vi "gps.vi"() -> ()   [LabVIEW 2020]
uses:
  <vilib>/Instr/_visa.llb/VISA Configure Serial Port (Instr).vi
panel:
  in  "COM":refnum<visa-resource-name>="COM7"
  in  "error in (no error)":errorcluster caption="에러 입력(에러 없음)"
  out "gga":string
  out "rmc":string
  out "vtg":string
  out "GGA cluster":T1
  out "RMC cluster":T2
  out "VTG cluster":T3
  out "TM_X(lat)":dbl format="%-#_10g M"
  out "TM_Y(long)":dbl format="%-#_10g M"
  out "Heading_T":dbl
  out "Heading_M":dbl
  out "F9P_Data_GPGGA_Raw":string
  out "GPS_KHP":dbl
  out "TM Current":cluster{dbl[], dbl[]}[](array[cluster])
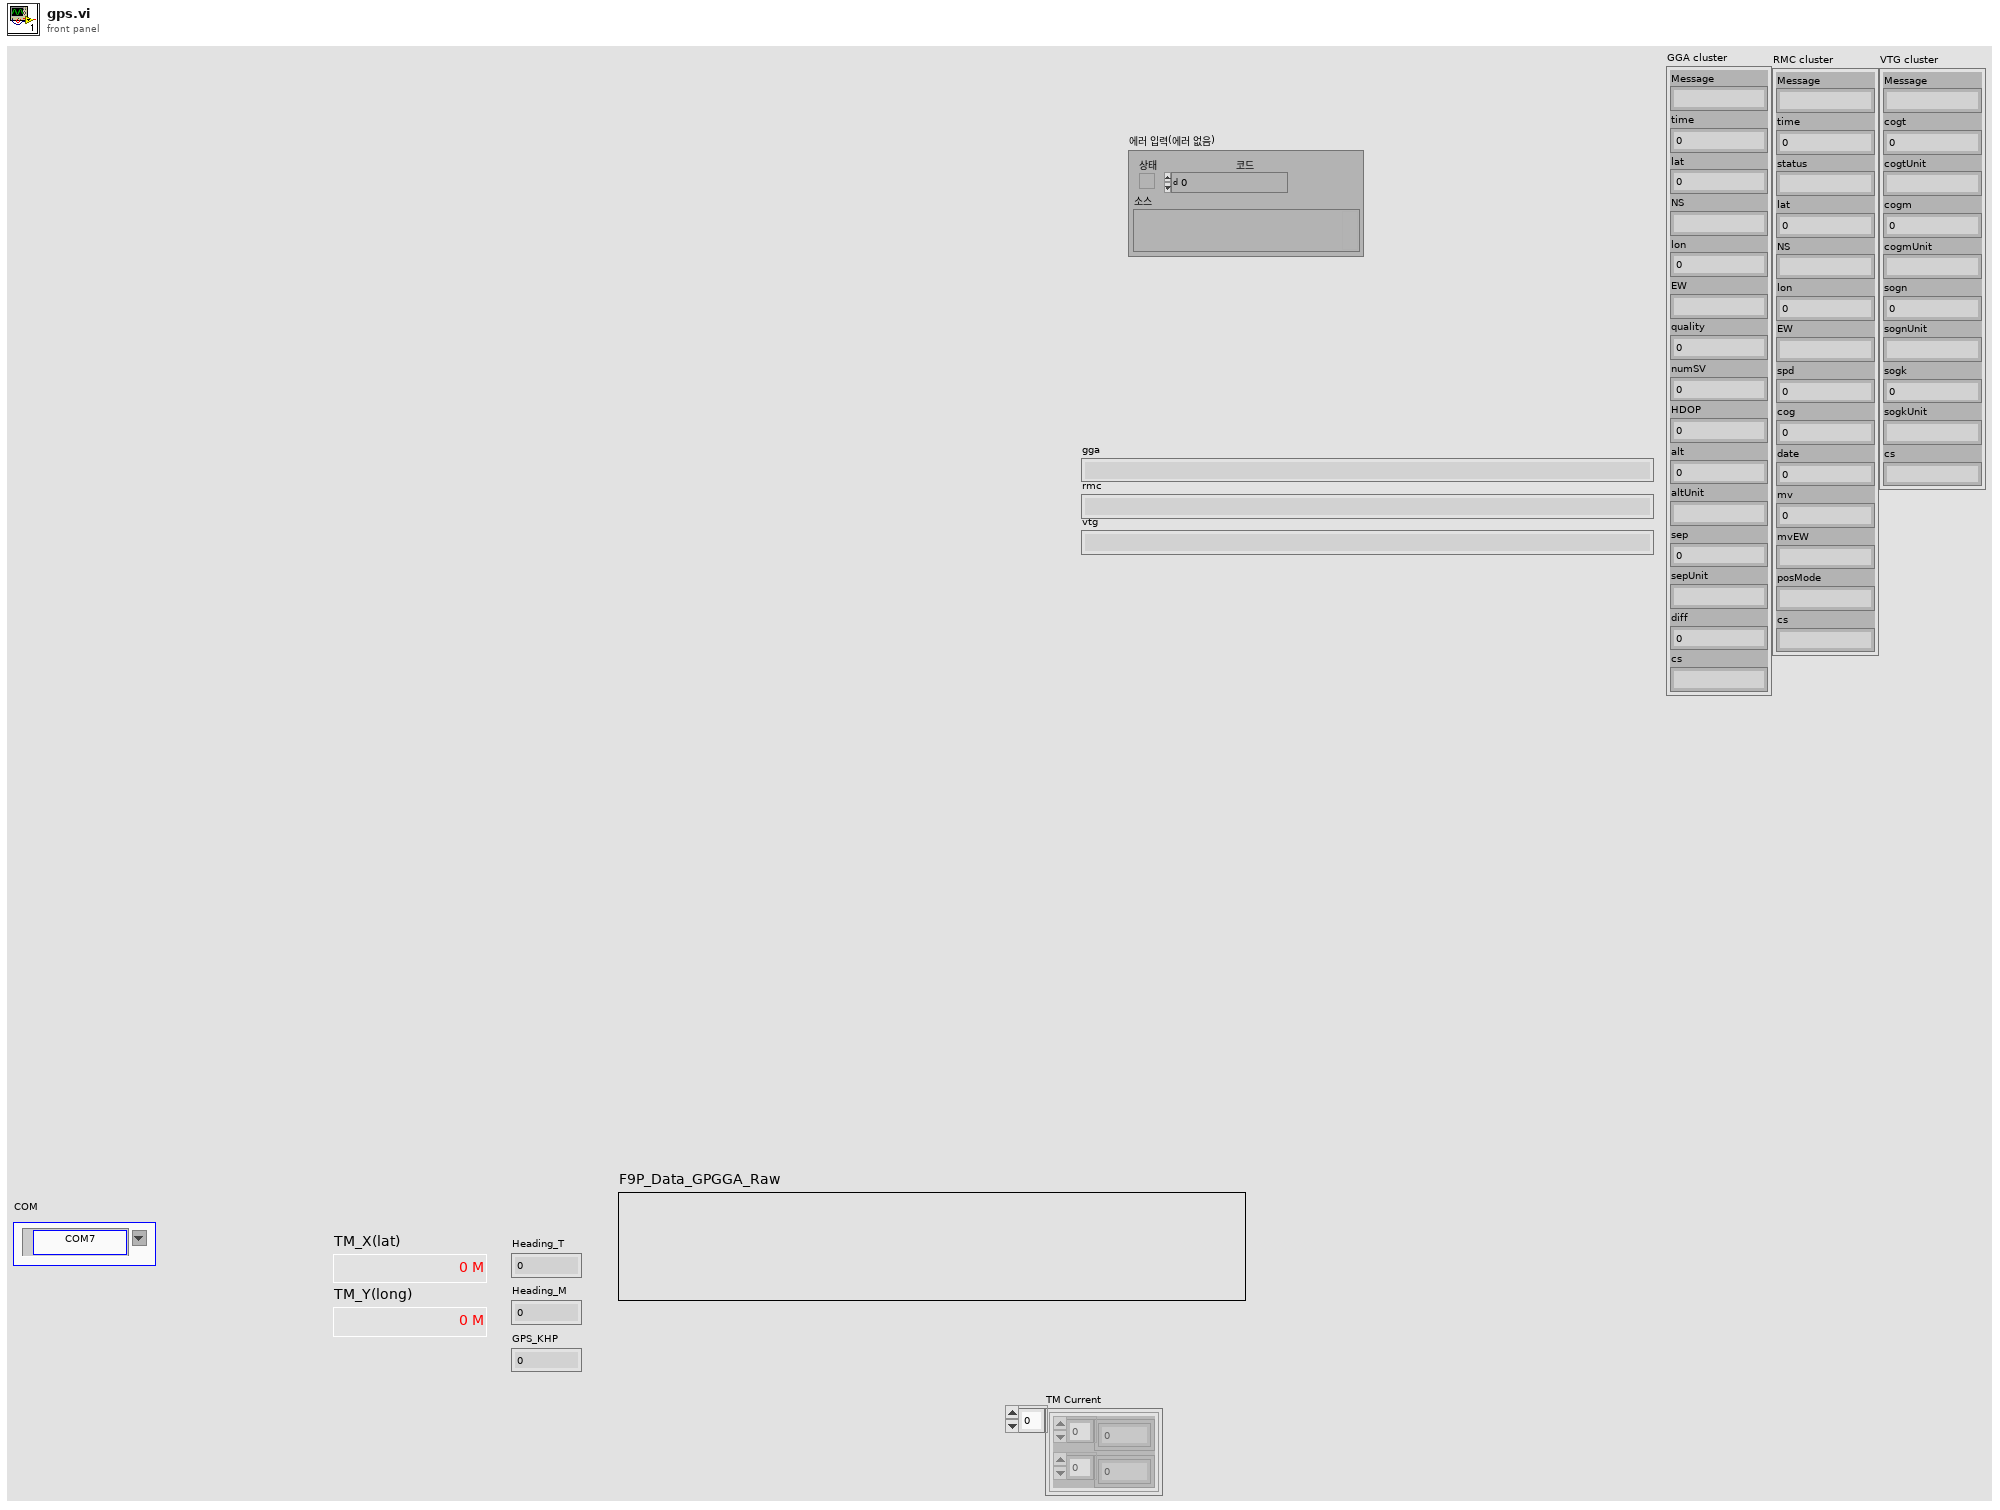
[diagram p1: front panel]
types:
  T1 = cluster{"Message":string, "time":dbl, "lat":dbl, "NS":string, "lon":dbl, "EW":string, "quality":u8, "numSV":u8, "HDOP":dbl, "alt":dbl, "altUnit":string, "sep":dbl, "sepUnit":string, "diff":i32, "cs":string}
  T2 = cluster{"Message":string, "time":dbl, "status":string, "lat":dbl, "NS":string, "lon":dbl, "EW":string, "spd":dbl, "cog":dbl, "date":u32, "mv":dbl, "mvEW":string, "posMode":string, "cs":string}
  T3 = cluster{"Message":string, "cogt":dbl, "cogtUnit":string, "cogm":dbl, "cogmUnit":string, "sogn":dbl, "sognUnit":string, "sogk":dbl, "sogkUnit":string, "cs":string}
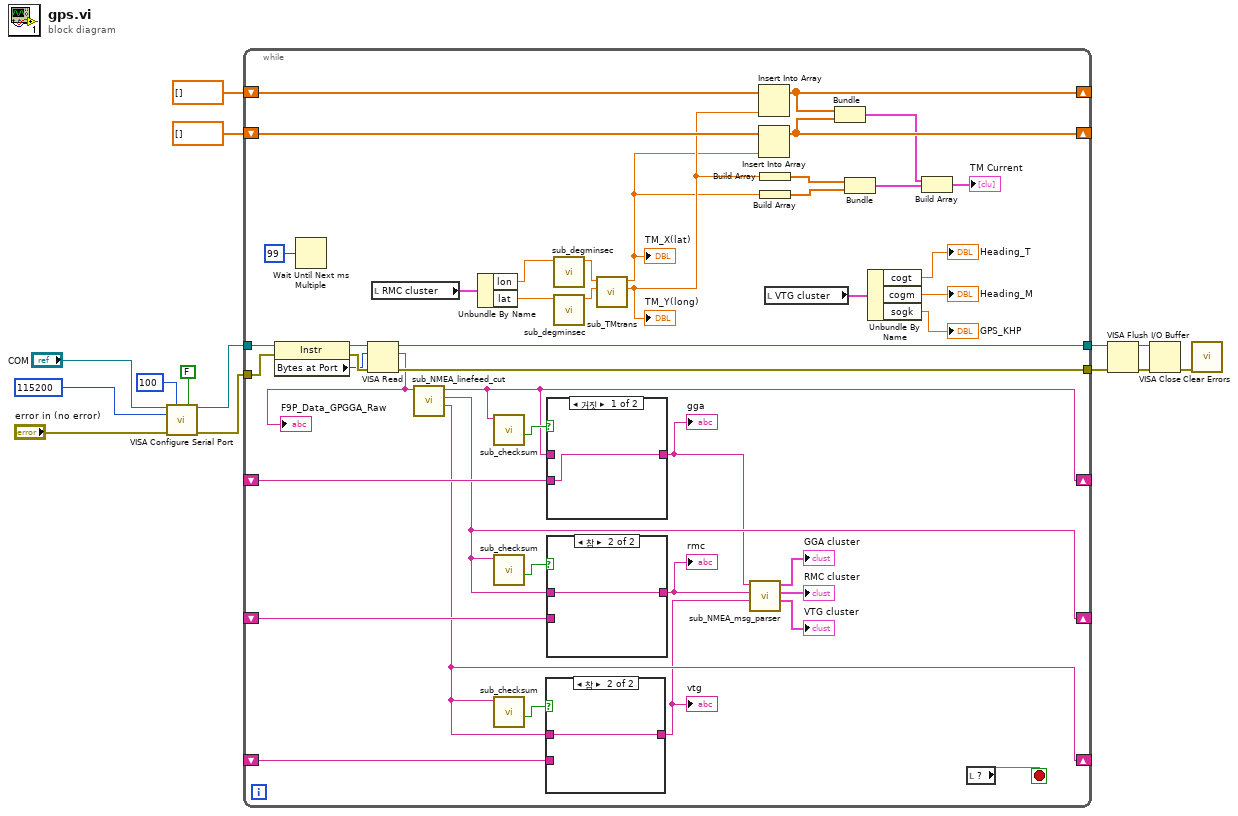
[diagram p0: block diagram]
diagram:
  n1 = call-poly "VISA Configure Serial Port"("VISA resource name"="COM", "timeout (10sec)"=u32 100, "Enable Termination\nChar (T)"=FALSE ("Enable Termination\nChar (T)"), "baud rate (9600)"=u32 115200, "error in (no error)"="error in (no error)") -> ("VISA resource name out"=w13:refnum<visa-resource-name>, "error out"=w12:errorcluster)  [unwired: 9 in]
  n2 = while {
    tunnel: w13 -> [w56]
    tunnel: w12 -> [w55]
    tunnel: [w58] -> w11
    tunnel: [w57] -> w10
    shift-right: [w45] -> _
    shift-left: _ -> [w50]
    shift-right: [w43] -> _
    shift-left: _ -> [w48]
    shift-right: [w44] -> _
    shift-left: _ -> [w46]
    shift-right: [w24] -> _
    shift-left: dbl[] [] -> [w26]
    shift-right: [w23] -> _
    shift-left: dbl[] [] -> [w25]
    stop <- w31 stop-if-true
    n3 = property class="Instr"(reference=w56, error in=w55) -> (reference out=w54:refnum<visa-resource-name>, error out=w53:errorcluster, "Bytes at Port"=w52:u32)
    n4 = Wait Until Next ms Multiple(millisecond multiple=u32 99 ("ms 배수")) -> ()  [unwired: 1 out]
    n5 = VISA Read(VISA resource name=w54, byte count=w52, error in (no error)=w53) -> (VISA resource name out=w58:refnum<visa-resource-name>, read buffer=w15:string, error out=w57:errorcluster)  [unwired: 1 out]
    "F9P_Data_GPGGA_Raw" <- w15
    n6 = local read "RMC cluster"() -> (w29:T2)
    n7 = call "sub_NMEA_linefeed_cut.vi"("GPS raw data buffer"=w15) -> ("GNVTG"=w44:string, "GNRMC"=w43:string, "GNGGA ($제거 문자열)"=w45:string)  [unwired: 8 in]
    n8 = Unbundle By Name(w29) -> ("lon"=w33:dbl, "lat"=w34:dbl)
    n9 = call "sub_checksum.vi"("NMEA String (~\\n이전)"=w45) -> ("equal?"=w51:bool)  [unwired: 6 in, 2 out]
    n10 = call "sub_checksum.vi"("NMEA String (~\\n이전)"=w43) -> ("equal?"=w49:bool)  [unwired: 6 in, 2 out]
    n11 = call "sub_checksum.vi"("NMEA String (~\\n이전)"=w44) -> ("equal?"=w47:bool)  [unwired: 6 in, 2 out]
    n12 = case shown="참" w47 {
      tunnel: [w60 w61] -> w40
      tunnel: w44 -> [_ w61]
      tunnel: w46 -> [w60 _]
      frame False {
      }
      frame True {
      }
    }
    "vtg" <- w40
    n13 = case shown="거짓" w51 {
      tunnel: [w64 w65] -> w42
      tunnel: w45 -> [_ w65]
      tunnel: w50 -> [w64 _]
      frame False {
      }
      frame True {
      }
    }
    "gga" <- w42
    n14 = case shown="참" w49 {
      tunnel: [w62 w63] -> w41
      tunnel: w43 -> [_ w63]
      tunnel: w48 -> [w62 _]
      frame False {
      }
      frame True {
      }
    }
    "rmc" <- w41
    n15 = call "sub_degminsec.vi"("경위도 (lon, lat)"=w33) -> ("도 (degree)"=w35:dbl)  [unwired: 9 in, 1 out]
    n16 = call "sub_degminsec.vi"("경위도 (lon, lat)"=w34) -> ("도 (degree)"=w36:dbl)  [unwired: 9 in, 1 out]
    n17 = call "sub_TMtrans.vi"("위도(lat)_Deg"=w36, "경도(lon)_Deg"=w35) -> ("TM_Y(long)"=w17:dbl, "TM_X(lat)"=w16:dbl)  [unwired: 8 in]
    "TM_X(lat)" <- w16
    "TM_Y(long)" <- w17
    n18 = call "sub_NMEA_msg_parser.vi"("VTG String ($이후~\\n이전)"=w40, "RMC String ($이후~\\n이전)"=w41, "GGA String ($이후~\\n이전)"=w42) -> ("VTG cluster"=→"VTG cluster":T3, "RMC cluster"=→"RMC cluster":T2, "GGA cluster"=→"GGA cluster":T1)  [unwired: 6 in]
    n19 = Insert Into Array(array=w26, new element=w17) -> (w24:dbl[])  [unwired: 1 in]
    n20 = Insert Into Array(array=w25, new element=w16) -> (w23:dbl[])  [unwired: 1 in]
    n21 = Build Array(w17) -> (w22:dbl[])
    n22 = Build Array(w16) -> (w21:dbl[])
    n23 = local read "VTG cluster"() -> (w32:T3)
    n24 = Bundle(w24, w23) -> (w19:cluster{dbl[], dbl[]})  [unwired: 1 in]
    n25 = Bundle(w22, w21) -> (w20:cluster{dbl[], dbl[]})  [unwired: 1 in]
    n26 = Unbundle By Name(w32) -> ("cogt"=→"Heading_T":dbl, "cogm"=→"Heading_M":dbl, "sogk"=→"GPS_KHP":dbl)
    n27 = Build Array(w19, w20) -> (→"TM Current":cluster{dbl[], dbl[]}[])
    n28 = local read item#-1() -> (w31)
  }
  n29 = VISA Flush I/O Buffer(VISA resource name=w11, error in (no error)=w10) -> (VISA resource name out=w9:refnum<visa-resource-name>, error out=w8:errorcluster)  [unwired: 1 in]
  n30 = VISA Close(VISA resource name=w9, error in (no error)=w8) -> (error out=w3:errorcluster)
  n31 = call <vilib>:"Clear Errors.vi"("error in (no error)"=w3) -> ()  [unwired: 5 in, 2 out]
